vi "ROI to 1D and 2D ROIs.vi"(11 "ROI Descriptor In":T1 {"Contours"."Type" items=["No Selection", "Point", "Line", "Rectangle", "Oval", "Polygon", "Freehand Region", "Annulus", "Unused2", "Unused3", "Broken Line", "Freehand Line", "Rotated Rectangle"]}) -> (2 "1D ROIs":T1 {"Contours"."Type" items=["No Selection", "Point", "Line", "Rectangle", "Oval", "Polygon", "Freehand Region", "Annulus", "Unused2", "Unused3", "Broken Line", "Freehand Line", "Rotated Rectangle"]}, 3 "2D ROIs":T1 {"Contours"."Type" items=["No Selection", "Point", "Line", "Rectangle", "Oval", "Polygon", "Freehand Region", "Annulus", "Unused2", "Unused3", "Broken Line", "Freehand Line", "Rotated Rectangle"]})   [LabVIEW 2014, in "POLARIS IMAQ Display.xctl"]
uses:
  POLARIS IMAQ Display.xctl
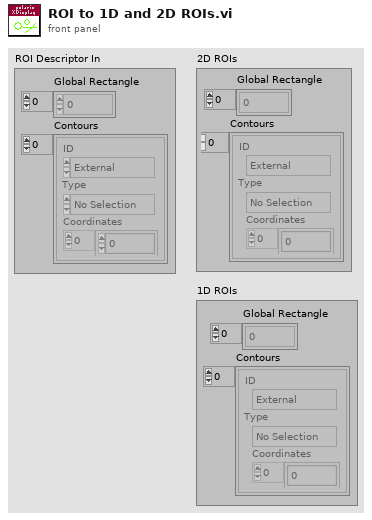
[diagram p1: front panel]
types:
  T1 = typedef "ROI Descriptor" = cluster{"Global Rectangle":i32[], "Contours":cluster{"ID":enum32{"External", "Internal"}, "Type":u32, "Coordinates":i32[]}[]}
  T2 = cluster{"ID":enum32{"External", "Internal"}, "Type":u32, "Coordinates":i32[]}[]
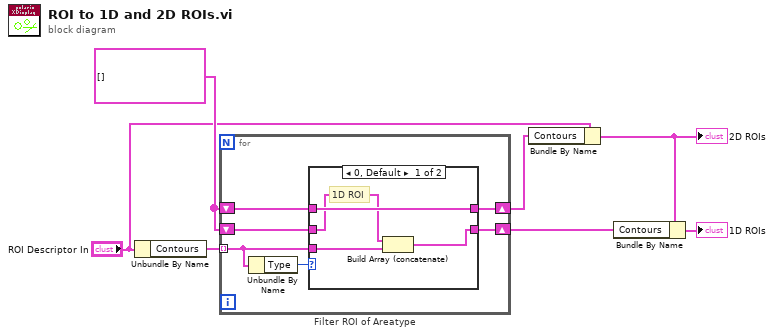
[diagram p0: block diagram]
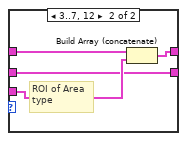
[diagram p2: hidden frame]
diagram:
  w5 = T2 []
  n1 = Unbundle By Name("ROI Descriptor In") -> ("Contours"=w6:T2)
  n2 = for "Filter ROI of Areatype" {
    tunnel: w6 -> [w12] mode=indexing
    shift-right: [w11] -> w7
    shift-left: w5 -> [w10]
    shift-right: [w8] -> w3
    shift-left: w5 -> [w9]
    n3 = Unbundle By Name(w12) -> ("Type"=w13:u32)
    n4 = case shown="0, Default" w13 {
      tunnel: w12 -> [w15 w21]
      tunnel: [w17 w20] -> w11
      tunnel: w10 -> [w17 w19]
      tunnel: w9 -> [w16 w18]
      tunnel: [w14 w18] -> w8
      frame 0, Default {
        # "1D ROI"
        n5 = Build Array (concatenate)(w16, w15) -> (w14:T2)
      }
      frame 3..7, 12 {
        # "ROI of Area\ntype"
        n6 = Build Array (concatenate)(w19, w21) -> (w20:T2)
      }
    }
  }
  n7 = Bundle By Name(cluster="ROI Descriptor In", "Contours"=w7) -> (w2:T1)
  "2D ROIs" <- w2
  n8 = Bundle By Name(cluster=w2, "Contours"=w3) -> (→"1D ROIs":T1)
